vi "VI_Modification_Dates.vi"   [LabVIEW 2011]
uses:
  Anemometry/Anemometry Sub Vis/Globals/Preference_global.vi
  Anemometry/Anemometry Sub Vis/Globals/Constants_global.vi
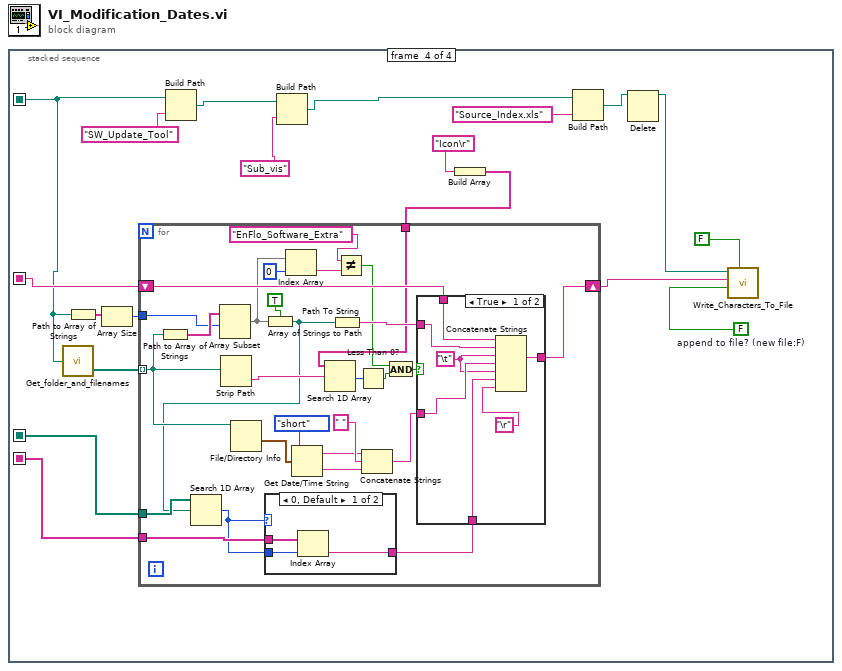
[diagram p0: block diagram]
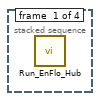
[diagram p2: hidden frame]
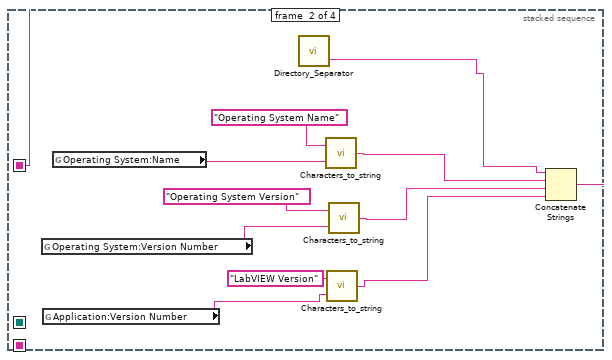
[diagram p3: hidden frame]
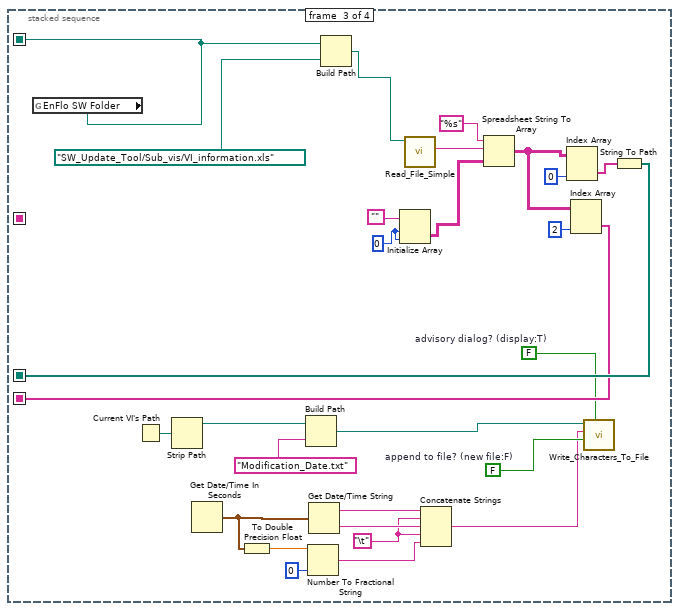
[diagram p4: hidden frame]
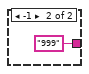
[diagram p5: hidden frame]
diagram:
  n1 = stacked-sequence {
    seq-local: [_ w5 _ _] -> [_ _ _ w51]
    seq-local: [_ _ w39 _] -> [_ _ _ w46]
    seq-local: [_ _ w29 _] -> [_ _ _ w48]
    seq-local: [_ _ w28 _] -> [_ _ _ w47]
    frame #0 {
      n2 = call "Run_EnFlo_Hub.vi"() -> ()  [unwired: 8 out]
    }
    frame #1 {
      n3 = global read "Preference_global.vi" "Operating System:Version Number"() -> (w3:string)
      n4 = global read "Preference_global.vi" "Application:Version Number"() -> (w2:string)
      n5 = global read "Preference_global.vi" "Operating System:Name"() -> (w4:string)
      n6 = call "Directory_Separator.vi"() -> ("Setup string"=w1:string)  [unwired: 2 out]
      n7 = call "Characters_to_string.vi"("Characters to write"=w4, "Label for characters"="Operating System Name") -> ("Output string"=w8:string)
      n8 = call "Characters_to_string.vi"("Characters to write"=w2, "Label for characters"="LabVIEW Version") -> ("Output string"=w6:string)
      n9 = call "Characters_to_string.vi"("Characters to write"=w3, "Label for characters"="Operating System Version") -> ("Output string"=w7:string)
      n10 = Concatenate Strings(w1, w8, w7, w6) -> (w5:string)
    }
    frame #2 {
      w17 = "\t"
      w20 = FALSE  # append to file? (new file:F)
      w21 = FALSE  # advisory dialog? (display:T)
      w36 = 0 ("Dimension Size")
      n11 = global read "Constants_global.vi" "EnFlo SW Folder"() -> (w39:path)
      n12 = Current VI's Path() -> (path=w25:path)
      n13 = Strip Path(path=w25) -> (stripped path=w24:path)  [unwired: 1 out]
      n14 = Get Date/Time In Seconds() -> (seconds since 1Jan1904=w14:timestamp)
      n15 = To Double Precision Float(number=w14) -> (double precision float=w15:dbl)
      n16 = Build Path(base path=w24, name or relative path="Modification_Date.txt") -> (appended path=w22:path)
      n17 = Number To Fractional String(number=w15, precision (6)=i16 0) -> (F-format string=w13:string)  [unwired: 2 out]
      n18 = Get Date/Time String(seconds (now)=w14) -> (date string=w19:string, time string=w18:string)  [unwired: 2 out]
      n19 = Build Path(base path=w39, name or relative path=path "SW_Update_Tool/Sub_vis/VI_information.xls") -> (appended path=w26:path)
      n20 = Initialize Array("", w36, w36) -> (w38:string[][])
      n21 = call "Read_File_Simple.vi"("Filename"=w26) -> ("string"=w35:string)  [unwired: 2 in, 7 out]
      n22 = Concatenate Strings(w19, w17, w18, w17, w13) -> (w12:string)
      n23 = Spreadsheet String To Array(format string="%s", spreadsheet string=w35, array type (2D Dbl)=w38) -> (array=w30:string[][])  [unwired: 1 out]
      n24 = Index Array(array=w30, index (col)=0 ("disabled index (col)")) -> (element=w32:string[])  [unwired: 1 in]
      n25 = Index Array(array=w30, index (col)=2 ("disabled index (col)")) -> (element=w28:string[])  [unwired: 1 in]
      n26 = call "Write_Characters_To_File.vi"("file path (dialog if empty)"=w22, "advisory dialog? (display:T)"=w21, "character string"=w12, "append to file? (new file:F)"=w20) -> ()  [unwired: 1 in, 4 out]
      n27 = String To Path(string=w32) -> (path=w29:path[])
    }
    frame #3 {
      w50 = FALSE  # append to file? (new file:F)
      n28 = call "Get_folder_and_filenames.vi"("file path (dialog if empty)"=w46) -> ("Files"=w58:path[])  [unwired: 1 out]
      n29 = Path to Array of Strings(0:w46) -> (2:w57:string[])  [unwired: 1 out]
      n30 = Array Size(array=w57) -> (size(s)=w56:i32)
      n31 = Build Path(base path=w46, name or relative path="SW_Update_Tool") -> (appended path=w42:path)
      n32 = Build Path(base path=w42, name or relative path="Sub_vis") -> (appended path=w43:path)
      n33 = Build Array("Icon\r") -> (w52:string[])
      n34 = for {
        tunnel: w58 -> [w81] mode=indexing
        tunnel: w56 -> [w85]
        shift-right: [w83] -> w55
        shift-left: w51 -> [w84]
        tunnel: w52 -> [w79]
        tunnel: w48 -> [w78]
        tunnel: w47 -> [w77]
        n35 = Path to Array of Strings(0:w81) -> (2:w86:string[])  [unwired: 1 out]
        n36 = Array Subset(array=w86, index=w85) -> (w66:string[])  [unwired: 1 in]
        n37 = Strip Path(path=w81) -> (name=w80:string)  [unwired: 1 out]
        n38 = File/Directory Info(path=w81) -> (last mod=w71:timestamp)  [unwired: 1 in, 6 out]
        n39 = Array of Strings to Path(0:w66, 1:TRUE ("relative")) -> (2:w67:path)
        n40 = Search 1D Array(1D array=w78, element=w67) -> (index of element=w69:i32)  [unwired: 1 out]
        n41 = case shown="0, Default" w69 {
          tunnel: w69 -> [w89 _]
          tunnel: w77 -> [w88 _]
          tunnel: [w87 "999"] -> w76
          frame 0, Default {
            n42 = Index Array(array=w88, index=w89) -> (element=w87:string)
          }
          frame -1 {
          }
        }
        n43 = Index Array(array=w66, index=0) -> (element=w63:string)
        n44 = Get Date/Time String(date format (0)=enum16{"short", "long", "abbreviated"}."short", seconds (now)=w71) -> (date string=w73:string, time string=w74:string)  [unwired: 1 out]
        n45 = Search 1D Array(1D array=w79, element=w80) -> (index of element=w68:i32)  [unwired: 1 out]
        n46 = Path To String(path=w67) -> (string=w82:string)
        n47 = Not Equal?(x="EnFlo_Software_Extra", y=w63) -> (x != y?=w61:bool)
        n48 = Less Than 0?(x=w68) -> (x < 0?=w62:bool)
        n49 = Concatenate Strings(w73, " " ("string"), w74) -> (w70:string)
        n50 = And(x=w61, y=w62) -> (x .and. y?=w60:bool)
        n51 = case shown="True" w60 {
          tunnel: w70 -> [w97 _]
          tunnel: w84 -> [w96 w98]
          tunnel: [w95 w98] -> w83
          tunnel: w82 -> [w94 _]
          tunnel: w76 -> [w92 _]
          frame True {
            w93 = "\t"
            n52 = Concatenate Strings(w96, w94, w93, w97, w93, w92, "\r") -> (w95:string)
          }
          frame False {
          }
        }
      }
      n53 = Build Path(base path=w43, name or relative path="Source_Index.xls") -> (appended path=w41:path)
      n54 = Delete(path (use dialog)=w41) -> (deleted path=w40:path)  [unwired: 1 in, 5 out]
      n55 = call "Write_Characters_To_File.vi"("file path (dialog if empty)"=w40, "advisory dialog? (display:T)"=FALSE, "character string"=w55, "append to file? (new file:F)"=w50) -> ()  [unwired: 1 in, 4 out]
    }
  }
